vi "NewtonsPSM_Conf_Harmonics.vi"(0 "VISA session":refnum<visa-resource-name>, 1 "Selected Harmonic (3)":i16=3 min=2 max=76 step=1, 2 "Harmonics Series Up to (64)":i16=64 min=2 max=64 step=1, 7 "THD Computation (single)":u16(ring) items=["Single", "Difference THD", "Series THD"], 11 "error in (no error)":errorcluster, 12 "Parameter (%)":u16(ring) items=["%", "dB"]) -> (4 "dup VISA session":refnum<visa-resource-name>, 15 "error out":errorcluster)   [LabVIEW 2025, in "NewtonsPSM1735.lvlib"]
doc: "This VI set the Harmonics Configuration for the PPA2530"
uses:
  NewtonsPSM1735.lvlib
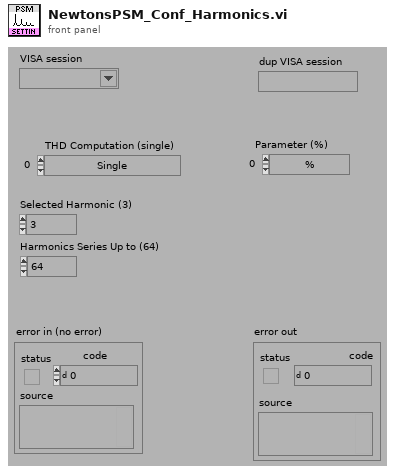
[diagram p1: front panel]
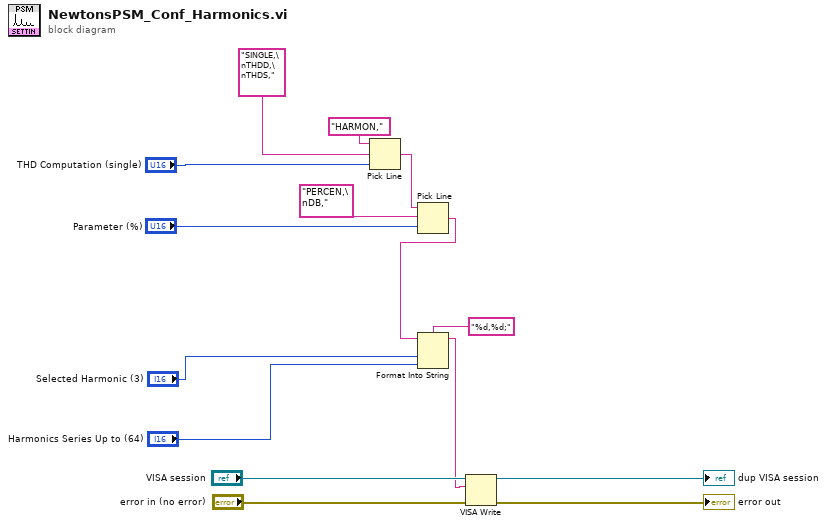
[diagram p0: block diagram]
diagram:
  n1 = Pick Line(string ("")="HARMON,", multi-line string="SINGLE,\nTHDD,\nTHDS,", line index="THD Computation (single)") -> (output string=w5:string)
  n2 = Pick Line(string ("")=w5, multi-line string="PERCEN,\nDB," ("chaîne multiligne"), line index="Parameter (%)") -> (output string=w2:string)
  n3 = Format Into String(format string="%d,%d;", initial string=w2, "Selected Harmonic (3)", "Harmonics Series Up to (64)") -> (resulting string=w1:string)  [unwired: 1 in, 1 out]
  n4 = VISA Write(VISA resource name="VISA session", write buffer=w1, error in (no error)="error in (no error)") -> (VISA resource name out=→"dup VISA session":refnum<visa-resource-name>, error out=→"error out":errorcluster)  [unwired: 1 out]
